vi "Elevator Control Loop - Motion Profile.vi"() -> ()   [LabVIEW 2014, in "Elevator System.lvlib"]
uses:
  Elevator System.lvlib
  <vilib>/Rock Robotics/WPI/MotorControl/WPI_MotorControlDeviceRef.ctl
  <vilib>/Rock Robotics/WPI/MotorControl/WPI_MotorControlType.ctl
  <vilib>/Rock Robotics/SystemInterfaces/Typedef/FPGA_TypedefDigitalModule.ctl
  <vilib>/Rock Robotics/SystemInterfaces/DIO/FPGA_DIOPWMChannel.ctl
  <vilib>/Rock Robotics/WPI/PWM/WPI_PWMDeadband.ctl
  <vilib>/Rock Robotics/WPI/CAN/Jaguar/SubVIs/WPI_CANJaguar_ControlMode.ctl
  <vilib>/Rock Robotics/WPI/CAN/TalonSRX/WPI_CANTalonSRX_APIControlMode.ctl
  <vilib>/Rock Robotics/WPI/PWM/WPI_PWMTransform_ConPane.ctl
  <vilib>/Platform/TimedLoop/XDataNode/timing_clust.ctl
  <vilib>/Platform/TimedLoop/XDataNode/nitl_modes.ctl
  <vilib>/Platform/TimedLoop/XDataNode/wakeup.ctl
  Typedef/FGVAction.ctl
  <vilib>/addons/control/pid/pid.llb/PID (DBL).vi
  SimulatorVIs/Simulation Input Global.vi
  <vilib>/platform/TimedLoop/XDataNode/XDataNode.xnode
  <vilib>/addons/control/pid/NI_PID_pid.lvlib
  <vilib>/Platform/TimedLoop/XDataNode/XDNodeRunTimeDep.lvlib
panel:
  in  "G Constant":dbl
  in  "FeedForward Kv":dbl=0.1
  in  "Max Velocity":dbl=100.0
  in  "Max Acceleration":dbl=100.0
  out "Plant Input":dbl(graph)
  in  "output range":cluster{"output high":dbl, "output low":dbl}={"output high"=1.0, "output low"=-1.0} {"output low" format="%.2f"; "output high" format="%.2f"}
  in  "PID gains":T1 {"derivative time (Td, min)" format="%.3f"; "integral time (Ti, min)" format="%.3f"; "proportional gain (Kc)" format="%.3f"}
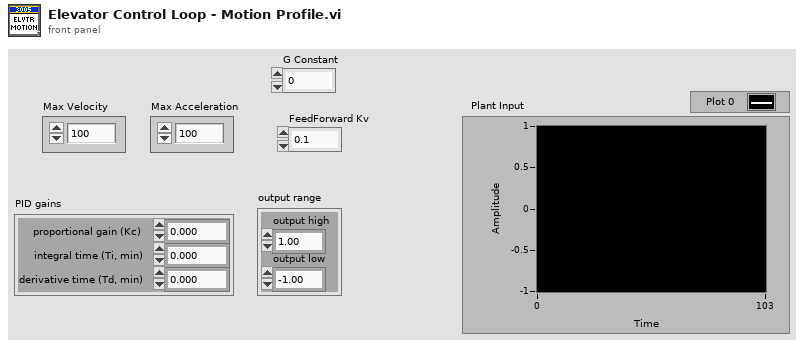
[diagram p1: front panel]
types:
  T1 = cluster{"proportional gain (Kc)":dbl, "integral time (Ti, min)":dbl, "derivative time (Td, min)":dbl}
  T2 = typedef "WPI_MotorControlDeviceRef.ctl" = cluster{"DeviceStatus":errorcluster, "Type":T3, "PWM":cluster{"Controller":T4, "PWM Channel":T5, "DeadBand":T6}, "CAN":cluster{"Device Number":u8, "Control Mode":T7, "Semaphore":T8, "Max Vout":dbl, "TalonSRX Control Mode":T9}, "Invert":bool, "TransformRef":T10, "InvTransformRef":T10}
  T3 = typedef "WPI_MotorControlType.ctl" = enum16{"PWM", "CAN", "CANTalonSRX"}
  T4 = typedef "FPGA_TypedefDigitalModule.ctl" = enum16{"Controller 1"}
  T5 = typedef "FPGA_DIOPWMChannel.ctl" = enum8{"PWM 0", "PWM 1", "PWM 2", "PWM 3", "PWM 4", "PWM 5", "PWM 6", "PWM 7", "PWM 8", "PWM 9", "PWM MXP 0", "PWM MXP 1", "PWM MXP 2", "PWM MXP 3", "PWM MXP 4", "PWM MXP 5", "PWM MXP 6", "PWM MXP 7", "PWM MXP 8", "PWM MXP 9", "Invalid"}
  T6 = typedef "WPI_PWMDeadband.ctl" = cluster{"Name":string, "maxPositivePwm":i32, "minPositivePwm":i32, "centerPwm":i32, "maxNegativePwm":i32, "minNegativePwm":i32, "angularRange":u16}
  T7 = typedef "WPI_CANJaguar_ControlMode.ctl" = enum8{"Percent VBus", "Current", "Speed", "Position", "Voltage"}
  T8 = typedef "Semaphore RefNum" = refnum<k1>
  T9 = typedef "WPI_CANTalonSRX_APIControlMode.ctl" = enum8{"Percent VBus", "Speed", "Position", "Slave", "Unchanged / Invalid"}
  T10 = typedef "WPI_PWMTransform_ConPane.ctl" = refnum<vi>
  T11 = cluster{"Setpoint":dbl, "notifier out":refnum<notifier>, "Output":dbl, "DriveMotor":T2, "Position":dbl, "SP Profile":cluster{"Position":dbl[], "Velocity":dbl[], "Time":dbl[]}, "Counter":i64}
  T12 = typedef "XDNodeRunTimeDep.lvlib/timing_clust.ctl" = cluster{"Expected End [f-1]":u64, "Actual End [f-1]":u64, "Finished Late? [f-1]":bool, "Expected End [i-1]":u64, "Actual End [i-1]":u64, "Finished Late? [i-1]":bool, "Expected Start [i]":u64, "Actual Start [i]":u64, "Expected Start [f]":u64, "Actual Start [f]":u64, "Source Name":string, "Structure Name":string, "Period":i64, "Deadline":i64, "Offset":i64, "Start":i64, "Priority":i32, "Timeout":i32, "Mode":T13, "Wakeup Reason":T14, "Error":errorcluster, "Source Type":string, "Secondary Source Type":string, "Global End Time":u64, "Global Start Time":u64, "Frame Duration":u64, "Iteration Duration":u64, "Assigned CPU":i32, "I/O Scan Engine Mode":u32}
  T13 = typedef "XDNodeRunTimeDep.lvlib/nitl_modes.ctl" = enum32{"No Change", "Process missed periods, maintain original phase", "Discard missed periods, maintain original phase", "Process missed periods, ignore original phase", "Discard missed periods, ignore original phase"}
  T14 = typedef "XDNodeRunTimeDep.lvlib/wakeup.ctl" = enum32{"Normal", "Aborted", "Asynchronous wakeup", "Timing source error", "Timed loop error", "Timeout"}
  T15 = typedef "Elevator System.lvlib/FGVAction.ctl" = enum16{"get", "set"}
  T16 = cluster{"Position":dbl[], "Velocity":dbl[], "Time":dbl[]}
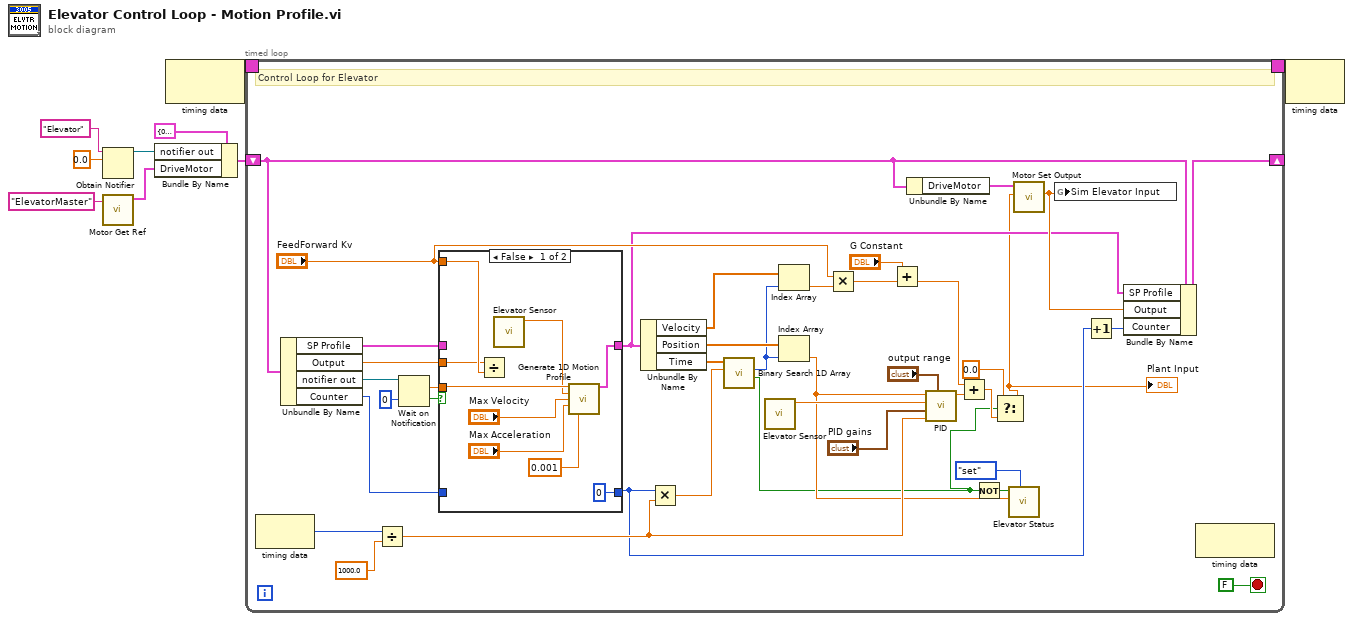
[diagram p0: block diagram]
diagram:
  n1 = Obtain Notifier(name (unnamed)="Elevator", notification data type=0.0 ("Setpoint")) -> (notifier out=w7:refnum<notifier>)  [unwired: 2 in, 2 out]
  n2 = call "Motor Get Ref.vi"("refnum name"="ElevatorMaster") -> ("MotorControlDevRef"=w4:T2)  [unwired: 10 in]
  n3 = Bundle By Name(cluster=T11 {"Setpoint"=0.0, "notifier out"=refnum, "Output"=0.0, "DriveMotor"={"DeviceStatus"={"status"=FALSE, "code"=0, "source"=""}, "Type"=enum."PWM", "PWM"={"Controller"=enum."Controller 1", "PWM Channel"=enum."Invalid", "DeadBand"={"Name"="", "maxPositivePwm"=0, "minPositivePwm"=0, "centerPwm"=0, "maxNegativePwm"=0, "minNegativePwm"=0, "angularRange"=0}}, "CAN"={"Device Number"=0, "Control Mode"=enum."Percent VBus", "Semaphore"=refnum, "Max Vout"=12.0, "TalonSRX Control Mode"=enum."Percent VBus"}, "Invert"=FALSE, "TransformRef"=refnum, "InvTransformRef"=refnum}, "Position"=0.0, "SP Profile"={"Position"=[], "Velocity"=[], "Time"=[]}, "Counter"=0}, "notifier out"=w7, "DriveMotor"=w4) -> (w8:T11)
  n4 = node-c288() -> (w2:T12)  [unwired: 1 in]
  n5 = timed-loop {
    shift-right: [w46] -> _
    shift-left: w8 -> [w38]
    timing: w2 -> [_]
    timing-out: [_] -> w1
    stop <- FALSE stop-if-true
    # "Control Loop for Elevator"
    n6 = node-c288() -> (w31:i64)  [unwired: 1 in]
    n7 = Unbundle By Name(w38) -> ("SP Profile"=w39:T16, "Output"=w41:dbl, "notifier out"=w47:refnum<notifier>, "Counter"=w33:i64)
    n8 = Divide(x=w31, y=1000.0) -> (x/y=w25:dbl)
    n9 = Wait on Notification(notifier=w47, timeout in ms (-1)=0) -> (notification=w42:dbl, timed out?=w43:bool)  [unwired: 2 in, 2 out]
    n10 = case shown="False" w43 {
      tunnel: w42 -> [w53 _]
      tunnel: "FeedForward Kv" -> [w58 _]
      tunnel: w41 -> [w57 _]
      tunnel: w39 -> [_ w62]
      tunnel: [w56 w62] -> w18
      tunnel: w33 -> [_ w61]
      tunnel: [i64 0 ("Counter") w61] -> w19
      frame False {
        # "New SP Given"
        n11 = Divide(x=w57, y=w58) -> ()  [unwired: 1 out]
        n12 = call "Elevator Sensor.vi"() -> ("Value"=w52:dbl)  [unwired: 10 in, 1 out]
        n13 = call "Generate 1D Motion Profile.vi"("Target Position"=w53, "Initial Position (0)"=w52, "Max Velocity"="Max Velocity", "Max Acceleration"="Max Acceleration", "resolution m (.001)"=0.001) -> ("Time Plot"=w56:T16)  [unwired: 8 in, 2 out]
      }
      frame True {
      }
    }
    n14 = Unbundle By Name(w18) -> ("Velocity"=w29:dbl[], "Position"=w28:dbl[], "Time"=w34:dbl[])
    n15 = Multiply(x=w19, y=w25) -> (x*y=w30:dbl)
    n16 = call "Binary Search 1D Array.vi"("element"=w30, "1D array sorted"=w34) -> ("Path Complete?"=w12:bool, "index"=w27:i32)  [unwired: 7 in, 1 out]
    n17 = call "Elevator Sensor.vi"() -> ("Value"=w26:dbl)  [unwired: 10 in, 1 out]
    n18 = Index Array(array=w29, index=w27) -> (element=w23:dbl)
    n19 = Index Array(array=w28, index=w27) -> (element=w14:dbl)
    n20 = Multiply(x="FeedForward Kv", y=w23) -> (x*y=w21:dbl)
    n21 = Add(x="G Constant", y=w21) -> (x+y=w16:dbl)
    n22 = Unbundle By Name(w38) -> ("DriveMotor"=w44:T2)
    n23 = call-poly <vilib>:"PID.vi"("output range"="output range", "dt (s)"=w25, "PID gains"="PID gains", "process variable"=w26, "setpoint"=w14) -> ("output"=w24:dbl)  [unwired: 5 in, 1 out]
    n24 = Add(x=w16, y=w24) -> (x+y=w17:dbl)
    n25 = Not(x=w12) -> (.not. x?=w10:bool)
    n26 = Select(t=0.0, s=w12, f=w17) -> (s? t:f=w13:dbl)
    "Plant Input" <- w13
    n27 = call "Elevator Status.vi"("Action"=FGVAction."set", "Input"=w14, "Moving? (F)"=w10) -> ()  [unwired: 6 in, 3 out]
    n28 = call "Motor Set Output.vi"("output"=w13, "DriveMotor"=w44) -> ("Motor Output"=w40:dbl)  [unwired: 9 in]
    n29 = global write "Simulation Input Global.vi" "Sim Elevator Input"(w40) -> ()
    n30 = Increment(x=w19) -> (x+1=w20:i64)
    n31 = Bundle By Name(cluster=w38, "SP Profile"=w18, "Output"=w40, "Counter"=w20) -> (w46:T11)
    n32 = node-c288() -> ()  [unwired: 1 in, 1 out]
  }
  n33 = node-c288(w1) -> ()  [unwired: 1 out]
